vi "WILT Update Aisle of Records.vi"   [LabVIEW 2016]
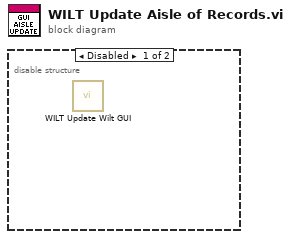
[diagram p0: block diagram]
diagram:
  n1 = disable-structure shown="Disabled" {
    frame Disabled {
      n2 = call "WILT Update Wilt GUI.vi"() -> ()  [unwired: 13 in, 3 out]
    }
    frame Enabled {
    }
  }
